vi "Populate Subpanels.vi"(8 "error in (no error)":errorcluster, 9 "View Labels (optional)":string[](array[string]), 10 "Views":refnum<class "Message Enqueuer.lvclass">[](array[class]), 11 "IViewManager In":refnum<class "IViewManager.lvclass">) -> (0 "error out":errorcluster, 3 "IViewManager Out":refnum<class "IViewManager.lvclass">)   [LabVIEW 2017, in "IViewManager.lvlib" / "IViewManager.lvclass"]
doc: "<License>\nCopyright © 2017 Composed Systems, LLC | All rights reserved\nwww.composed.io\n\nAuthor: Ethan Stern <ethan.stern@composed.io>\n\nThis software is provided \"AS IS\" WITHOUT WARRANTIES, either express or implied, AND IS FOR EDUCATIONAL PURPOSES ONLY.\n</License>"
uses:
  IViewManager.lvclass
  <vilib>/ActorFramework/Message Enqueuer/Message Enqueuer.lvclass
  IViewManager.lvclass/IViewManager.ctl
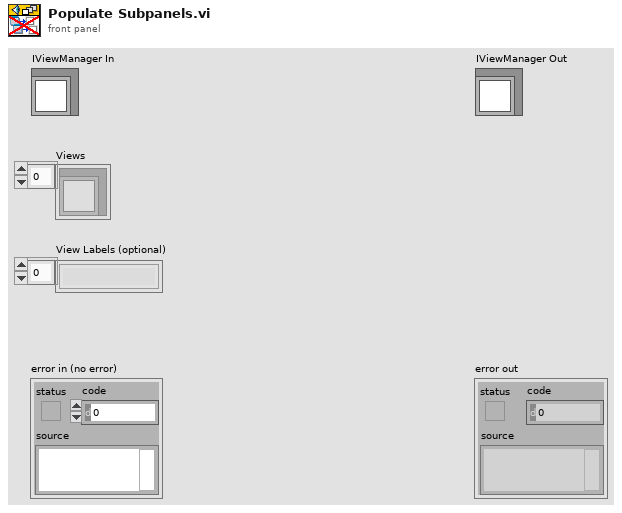
[diagram p1: front panel]
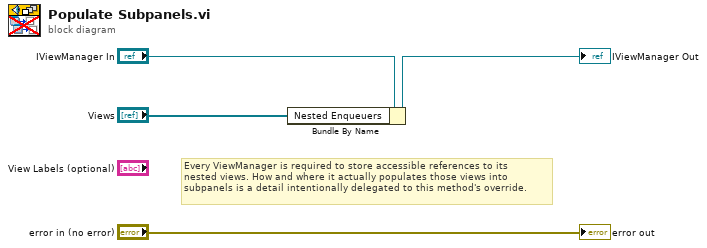
[diagram p0: block diagram]
diagram:
  # "Every ViewManager is required to store accessible references to its\nnested views. How and where it actually populates those views into\nsubpanels is a detail intentionally delegated to this method's override."
  n1 = Bundle By Name(cluster="IViewManager In", "Nested Enqueuers"="Views") -> (→"IViewManager Out":refnum<class "IViewManager.lvclass">)
  "error out" <- "error in (no error)"
